vi "SVL AC & DC Level (1 Ch SGL Array).vi"(9 "window":u16(ring)=8 items=["None ", "Hanning", "Hamming", "Blackman-Harris", "Exact Blackman", "Blackman", "Flat Top", "4 Term B-Harris ", "7 Term B-Harris", "Low Sidelobe"], 11 "scaled signal [EU]":sgl[](array[numeric])) -> (1 "DC level [EU]":dbl=nan format="%0.2f", 2 "AC level [EU rms]":dbl=nan format="%.8f", 3 "AC signal [EU]":sgl[](array[numeric]))   [LabVIEW 2017]
doc: "Computes the AC level and DC level of a signal. Wire data to the <B>scaled signal [EU]</B> input to determine the polymorphic instance to use or manually select the instance."
uses:
  <vilib>/Analysis/baseanly.llb/Mean (DBL).vi
  <vilib>/Analysis/0measdsp.llb/Scaled Time Domain Window (DBL).vi
  <vilib>/Analysis/NI_AALBase.lvlib
  <vilib>/Analysis/NI_AALPro.lvlib
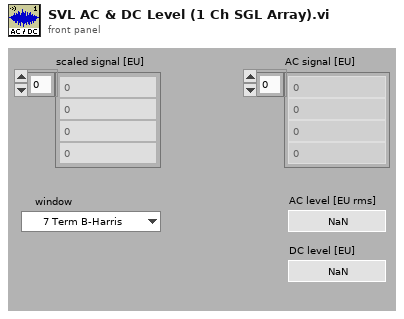
[diagram p1: front panel]
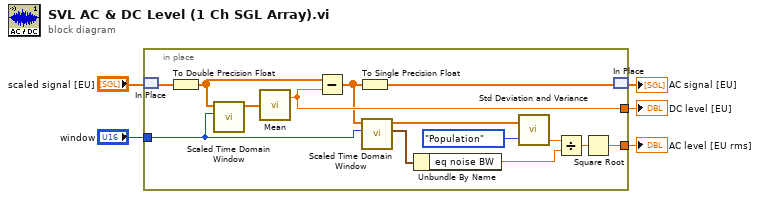
[diagram p0: block diagram]
diagram:
  n1 = in-place {
    in-place-border: [w19] -> w5
    in-place-border: "window" -> [w18]
    in-place-border: [w10] -> w3
    n2 = in-place-match #1("scaled signal [EU]") -> (w7:sgl[])
    n3 = To Double Precision Float(number=w7) -> (double precision float=w8:dbl[])
    n4 = call-poly <vilib>:"Scaled Time Domain Window.vi"("window"=w18, "X"=w8) -> ("Windowed X"=w14:dbl[])  [unwired: 7 in, 2 out]
    n5 = call-poly <vilib>:"Mean.vi"("X"=w14) -> ("mean"=w10:dbl)  [unwired: 1 out]
    n6 = Subtract(x=w8, y=w10) -> (x-y=w9:dbl[])
    n7 = To Single Precision Float(number=w9) -> (single precision float=w6:sgl[])
    n8 = call-poly <vilib>:"Scaled Time Domain Window.vi"("window"=w18, "X"=w9) -> ("window properties"=w11:cluster{"eq noise BW":dbl, "coherent gain":dbl}, "Windowed X"=w13:dbl[])  [unwired: 7 in, 1 out]
    n9 = Unbundle By Name(w11) -> ("eq noise BW"=w12:dbl)
    n10 = call <vilib>:"Std Deviation and Variance.vi"("X"=w13, "Weighting (Sample)"=enum16{"Sample", "Population"}."Population") -> ("variance"=w17:dbl)  [unwired: 2 out]
    n11 = Divide(x=w17, y=w12) -> (x/y=w15:dbl)
    n12 = Square Root(x=w15) -> (sqrt(x)=w19:dbl)
    n13 = in-place-match #1(w6) -> (→"AC signal [EU]":sgl[])
  }
  "AC level [EU rms]" <- w5
  "DC level [EU]" <- w3
